vi "roi_scratch_program.vi"() -> ()   [LabVIEW 2019]
uses:
  SampleCalibrationCalculationResults_cluster_typedef.ctl
  a6b3d2e8-befa-4aaa-a736-0ac2335bbd44.vi
  e0302028-5bfe-410e-abbb-8cfbcfc24c06.vi
  04559565-41ae-42aa-85bd-c458572823e8.vi
  <vilib>/Array/Sort 2D Array - Pop Stack.vi
  <vilib>/Array/Sort 2D Array - Push Stack.vi
  a6b3d2e8-befa-4aaa-a736-0ac2335bbd44.vi/0ef84ebb-a71d-453b-bf51-364b2a8100c2.vi
  a6b3d2e8-befa-4aaa-a736-0ac2335bbd44.vi/eded5715-ca70-42e2-b184-fcdb46cd780e.vi
  e0302028-5bfe-410e-abbb-8cfbcfc24c06.vi/4418a156-f814-4ade-9ace-40d5dcab888c.vi
  e0302028-5bfe-410e-abbb-8cfbcfc24c06.vi/000562a0-02a9-4d47-bc11-34049ac1e947.vi
  04559565-41ae-42aa-85bd-c458572823e8.vi/0594268f-122f-4dda-8abd-4fe50bdc6ae3.vi
  04559565-41ae-42aa-85bd-c458572823e8.vi/138f58bd-f8f8-424e-a1dc-8fd2d50bb075.vi
  <vilib>/vision/NI_Vision_Development_Module.lvlib
panel:
  out "x/y":dbl
  out "subarray 2":sgl[][](array[numeric])
  out "subarray":sgl[][](array[numeric])
  out "appended array":sgl[][](array[numeric])
  out "sorted 2D array":sgl[][](array[numeric])
  in  "ROI Size":dbl
  in  "N ROIs":dbl
  in  "Tab Control":enum32{"Page 1", "Page 2"}(tab)
  in  "Image 3":path
  out "Image 1":T1(plugin-control)
  out "Image 4":T1(plugin-control)
  in  "Image 2":path
  out "Calculation Results":T2
  in  "Calculate":bool
  in  "Next":bool
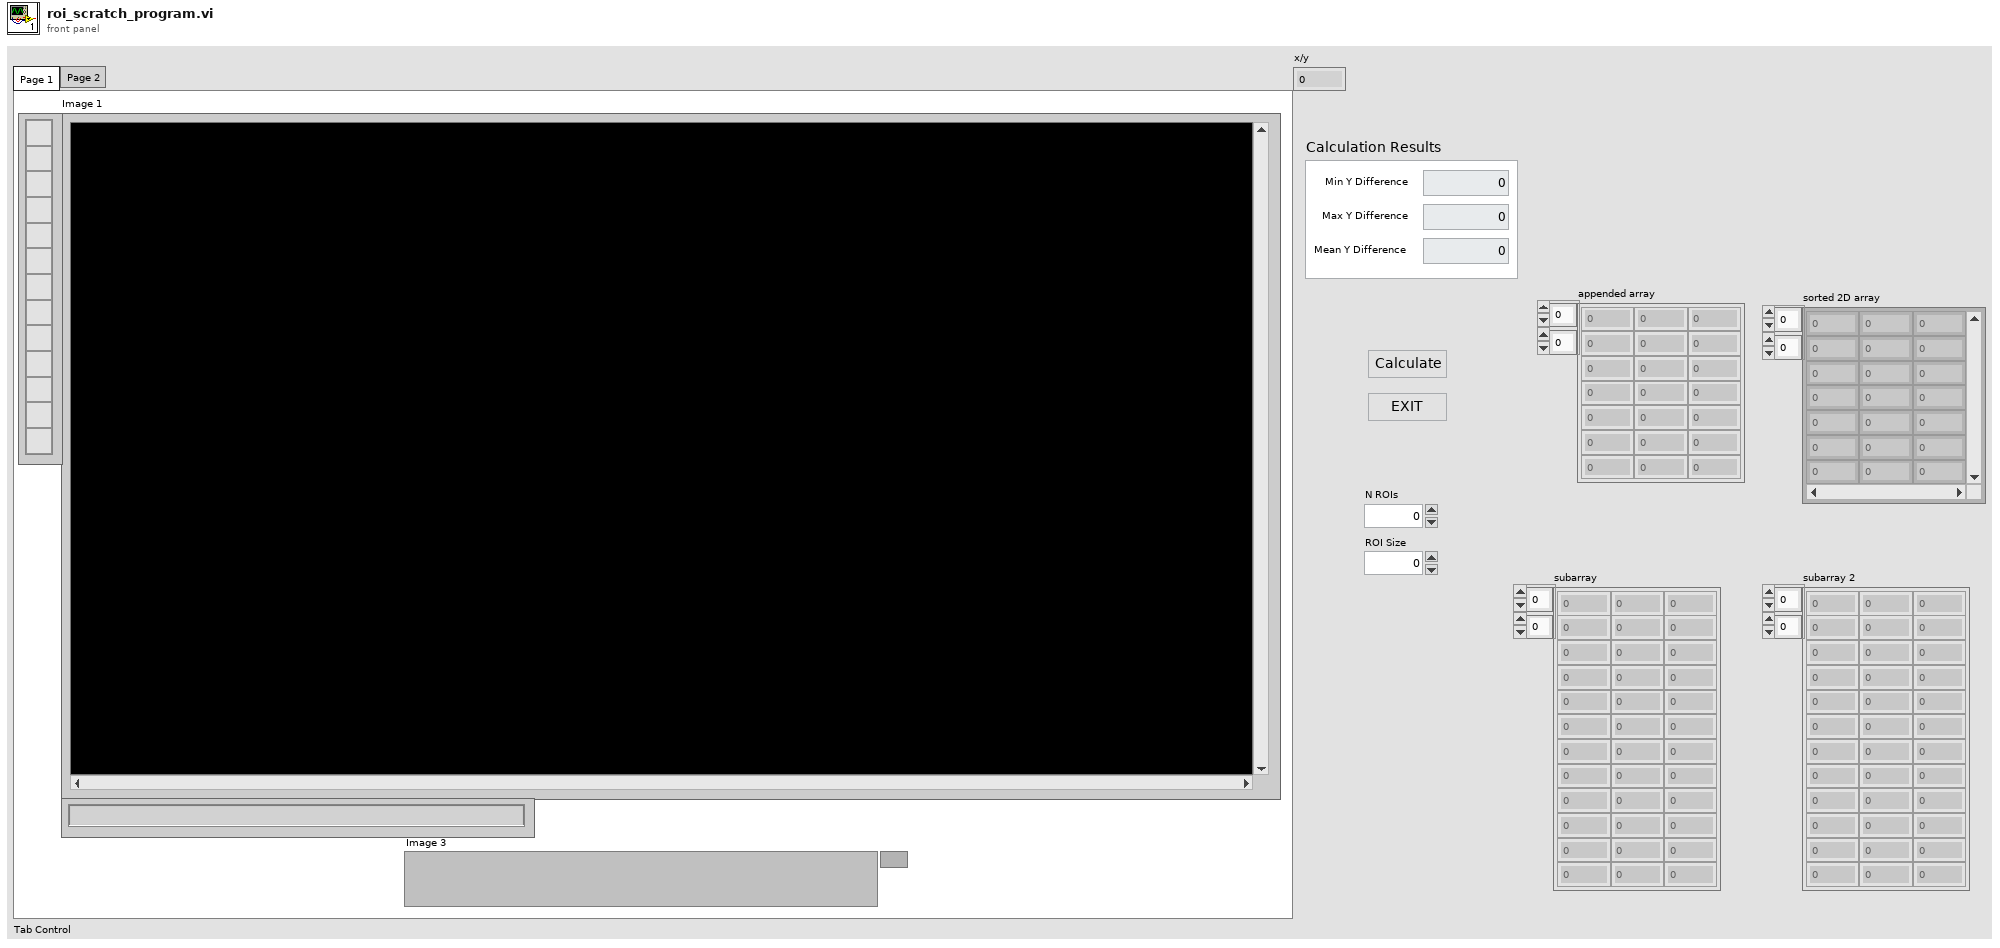
[diagram p1: front panel]
types:
  T1 = typedef "IMAQ Image.ctl" = refnum<image>
  T2 = typedef "SampleCalibrationCalculationResults_cluster_typedef.ctl" = cluster{"Mean Y Difference":dbl, "Max Y Difference":dbl, "Min Y Difference":dbl}
  T3 = typedef "Image Type" = u32
  T4 = cluster{"Global Rectangle":i32[], "Contours":cluster{"Contour Type":u32, "ROI Type":u32, "Points":i32[]}[]}
  T5 = cluster{"Contour Type":u32, "ROI Type":u32, "Points":i32[]}[]
  T6 = typedef "ROI Descriptor" = cluster{"Global Rectangle":i32[], "Contours":cluster{"ID":enum32{"External", "Internal"}, "Type":u32, "Coordinates":i32[]}[]}
  T7 = cluster{"Position":cluster{"X":sgl, "Y":sgl}, "Angle":dbl, "Major Radius":dbl, "Minor Radius":dbl, "Score":dbl}[]
  T8 = cluster{"Position":cluster{"X":sgl, "Y":sgl}, "Angle":dbl, "Major Radius":dbl, "Minor Radius":dbl, "Score":dbl}
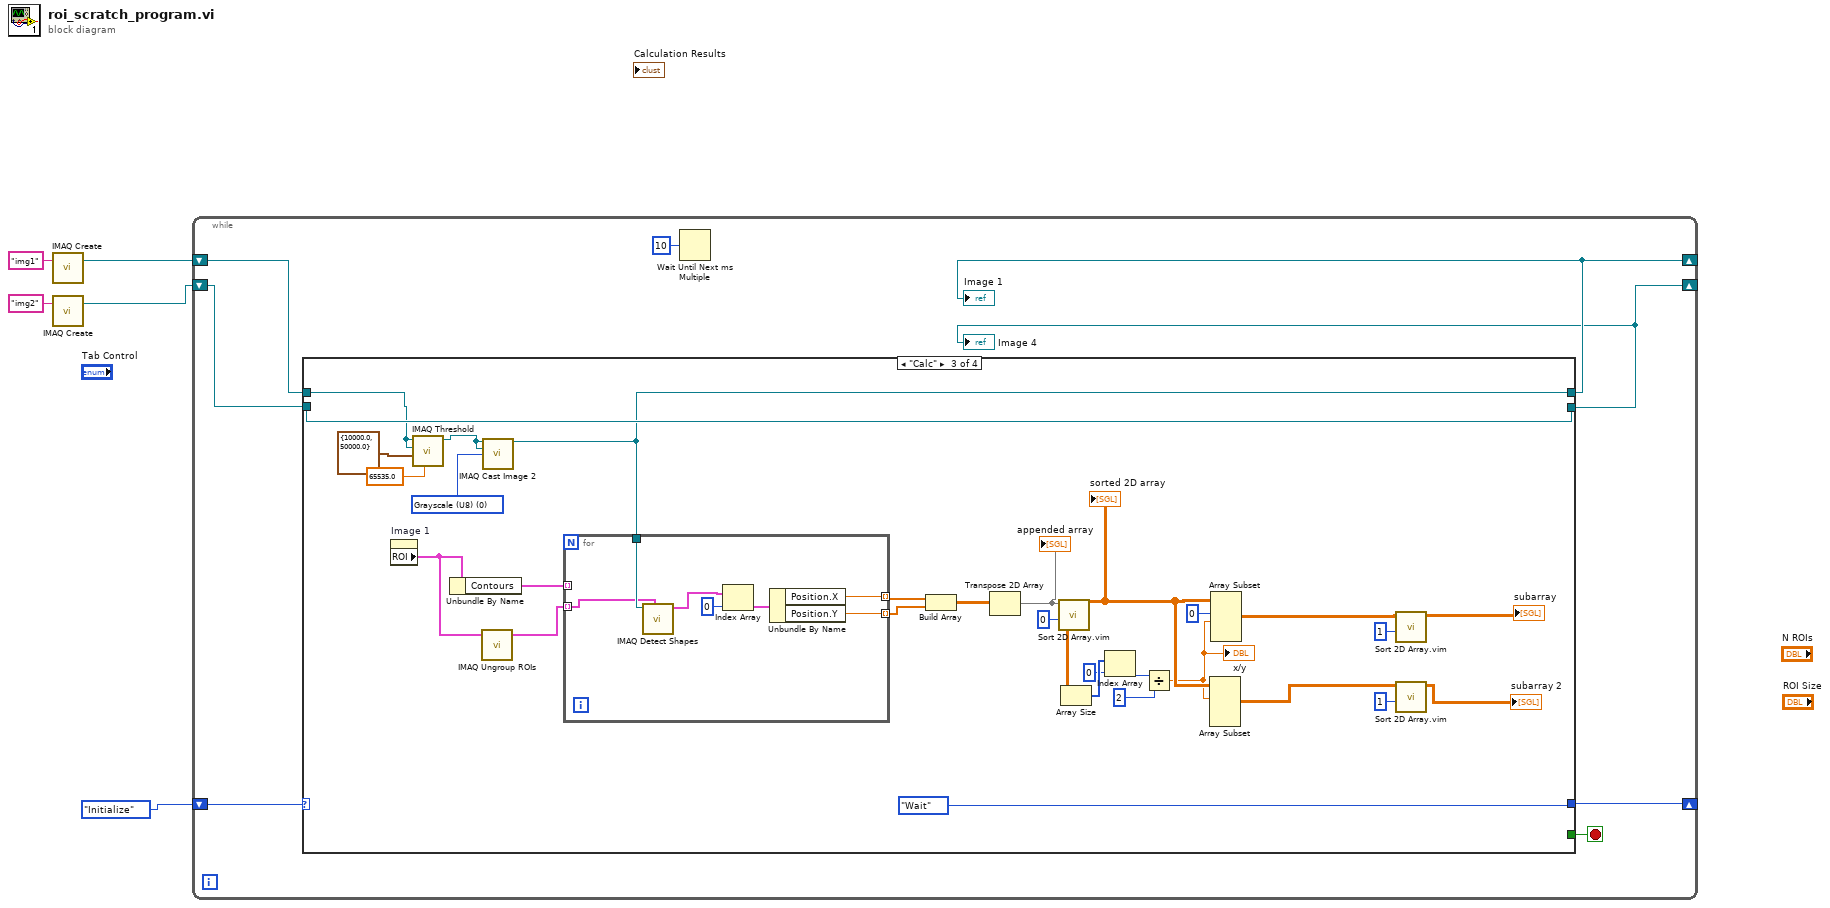
[diagram p0: block diagram]
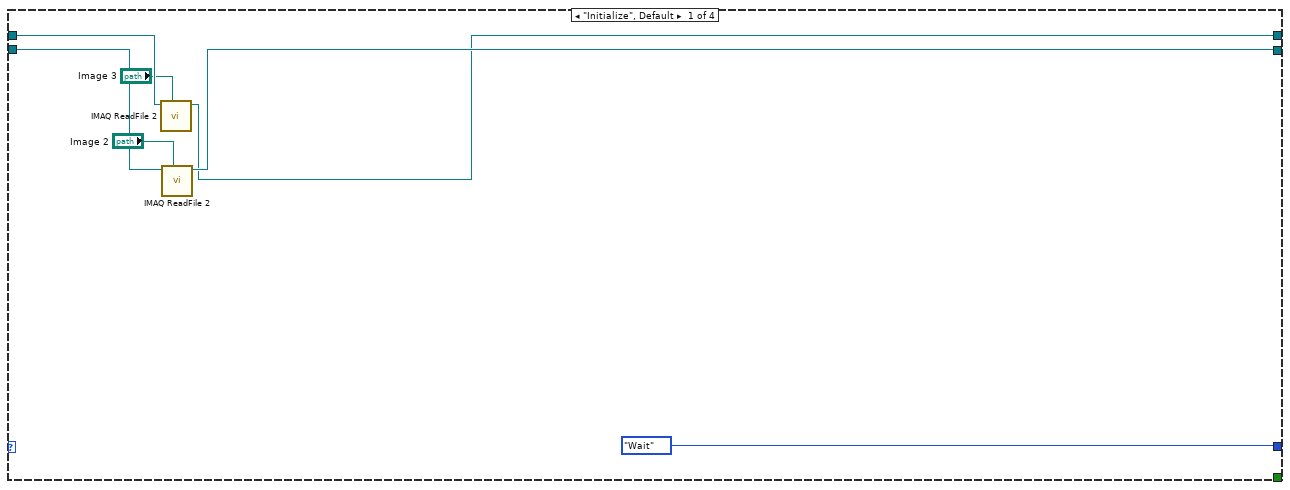
[diagram p2: hidden frame]
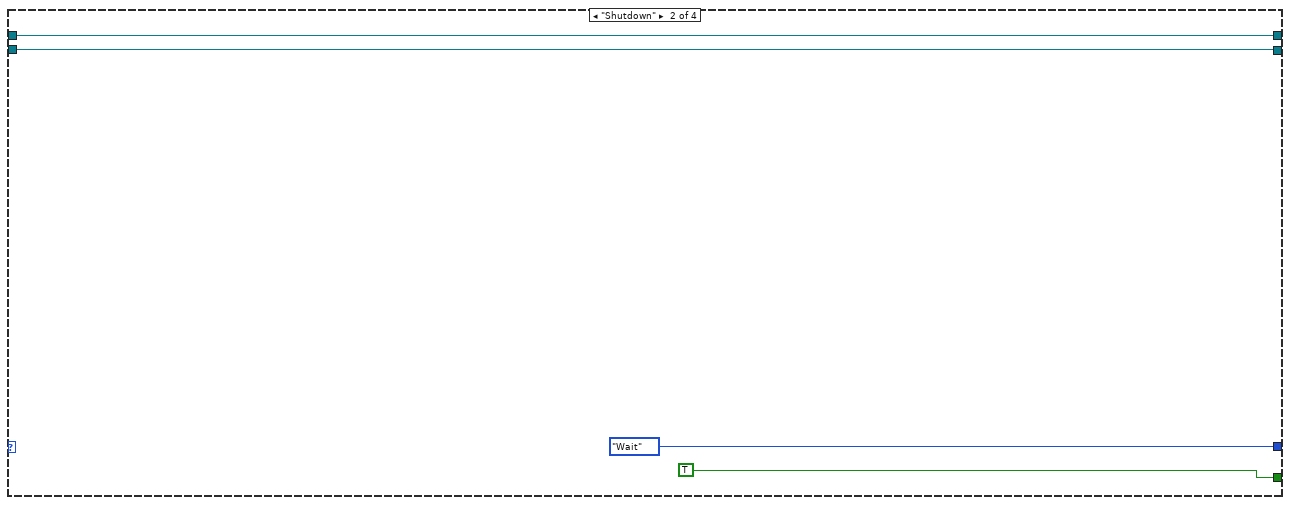
[diagram p3: hidden frame]
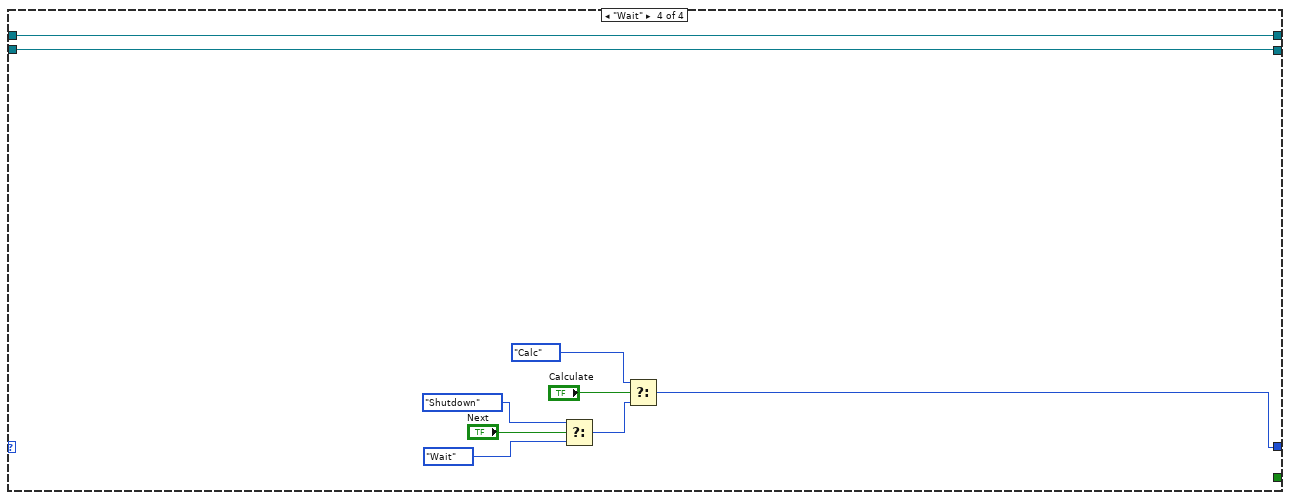
[diagram p4: hidden frame]
diagram:
  n1 = call "IMAQ Create"("Image Name"="img1") -> ("New Image"=w2:T1)  [unwired: 4 in, 1 out]
  n2 = call "IMAQ Create"("Image Name"="img2") -> ("New Image"=w1:T1)  [unwired: 4 in, 1 out]
  n3 = while {
    shift-right: [w12] -> _
    shift-left: enum16{"Initialize", "Shutdown", "Calc", "Wait"}."Initialize" -> [w13]
    shift-right: [w8] -> _
    shift-left: w2 -> [w10]
    shift-right: [w7] -> _
    shift-left: w1 -> [w9]
    stop <- w6 stop-if-true
    n4 = case shown="\"Calc\"" w13 {
      tunnel: [enum16{"Initialize", "Shutdown", "Calc", "Wait"}."Wait" enum16{"Initialize", "Shutdown", "Calc", "Wait"}."Wait" enum16{"Initialize", "Shutdown", "Calc", "Wait"}."Wait" w63] -> w12
      tunnel: w10 -> [w20 w23 w50 w62]
      tunnel: w9 -> [w19 w22 w52 w61]
      tunnel: [w14 w23 w45 w62] -> w8
      tunnel: [w16 w22 w52 w61] -> w7
      tunnel: [_ TRUE _ _] -> w6
      frame "Initialize", Default {
        n5 = call "IMAQ ReadFile 2"("File Path"="Image 3", "Image"=w20) -> ("Image Out"=w14:T1)  [unwired: 5 in, 4 out]
        n6 = call "IMAQ ReadFile 2"("File Path"="Image 2", "Image"=w19) -> ("Image Out"=w16:T1)  [unwired: 5 in, 4 out]
      }
      frame "Shutdown" {
      }
      frame "Calc" {
        w46 = T3 0 items=["Grayscale (U8)", "Grayscale (I16)", "Grayscale (SGL)", "Complex (CSG)", "RGB (U32)", "HSL (U32)", "RGB (U64)", "Grayscale (U16)"] ("Image Type")
        n7 = property on="Image 1" class="ImageControl"() -> ("ROI"=w44:T4)  [unwired: 2 in, 2 out]
        n8 = call "IMAQ Threshold"("Replace Value"=sgl 65535.0, "Range"=cluster{"Lower value":sgl, "Upper value":sgl} {"Lower value"=10000.0, "Upper value"=50000.0}, "Image Dst"=w50, "Image Src"=w50) -> ("Image Dst Out"=w47:T1)  [unwired: 6 in, 1 out]
        n9 = Unbundle By Name(w44) -> ("Contours"=w48:T5)
        n10 = call "IMAQ Ungroup ROIs"("ROI Descriptor"=w44) -> ("ROI Descriptors out"=w43:T6[])  [unwired: 3 in, 1 out]
        n11 = call "IMAQ Cast Image 2"("Image Src"=w47, "Image Dst"=w47, "Image Type"=w46) -> ("Image Dst Out"=w45:T1)  [unwired: 11 in, 1 out]
        n12 = for {
          tunnel: w48 -> [_] mode=indexing
          tunnel: w45 -> [w60]
          tunnel: [w56] -> w42 mode=indexing
          tunnel: [w55] -> w41 mode=indexing
          tunnel: w43 -> [w54] mode=indexing
          n13 = call-poly "IMAQ Detect Shapes"("ROI Descriptor"=w54, "Image"=w60) -> ("Ellipses"=w57:T7)  [unwired: 7 in, 2 out]
          n14 = Index Array(array=w57, index=0) -> (element=w58:T8)
          n15 = Unbundle By Name(w58) -> ("Position.X"=w56:sgl, "Position.Y"=w55:sgl)
        }
        n16 = Build Array(w42, w41) -> (w39:sgl[][])
        n17 = Transpose 2D Array(2D array=w39) -> (transposed array=w38:sgl[][])
        "appended array" <- w38
        n18 = call "Sort 2D Array.vim"("index"=0, "2D array"=w38) -> ("sorted 2D array"=w32:sgl[][])  [unwired: 8 in, 1 out]
        "sorted 2D array" <- w32
        n19 = Array Size(array=w32) -> (size(s)=w37:i32[])
        n20 = Index Array(array=w37, index=0) -> (element=w35:i32)
        n21 = Divide(x=w35, y=2) -> (x/y=w31:dbl)
        "x/y" <- w31
        n22 = Array Subset(array=w32, index (row)=w31) -> (w28:sgl[][])  [unwired: 3 in]
        n23 = Array Subset(array=w32, index (row)=0 ("index"), length (row)=w31) -> (w30:sgl[][])  [unwired: 2 in]
        n24 = call "Sort 2D Array.vim"("index"=1, "2D array"=w30) -> ("sorted 2D array"=→"subarray":sgl[][])  [unwired: 8 in, 1 out]
        n25 = call "Sort 2D Array.vim"("index"=1, "2D array"=w28) -> ("sorted 2D array"=→"subarray 2":sgl[][])  [unwired: 8 in, 1 out]
      }
      frame "Wait" {
        n26 = Select(t=enum16{"Initialize", "Shutdown", "Calc", "Wait"}."Shutdown", s="Next", f=enum16{"Initialize", "Shutdown", "Calc", "Wait"}."Wait") -> (s? t:f=w67:enum16{"Initialize", "Shutdown", "Calc", "Wait"})
        n27 = Select(t=enum16{"Initialize", "Shutdown", "Calc", "Wait"}."Calc", s="Calculate", f=w67) -> (s? t:f=w63:enum16{"Initialize", "Shutdown", "Calc", "Wait"})
      }
    }
    "Image 1" <- w8
    "Image 4" <- w7
    n28 = Wait Until Next ms Multiple(millisecond multiple=u32 10) -> ()  [unwired: 1 out]
  }
